vi "Fit Transform.vi"(7 "Type X":T1(ring), 8 "error in (no error)":errorcluster caption="entrée d'erreur (pas d'erreur)", 10 "X":string[][](array[string]), 11 "MissingIndicator.lvclass":refnum<class "MissingIndicator.lvclass">) -> (0 "error out":errorcluster caption="sortie d'erreur", 2 "Data":T2, 3 "MissingIndicator.lvclass":refnum<class "MissingIndicator.lvclass">)   [LabVIEW 2020, in "MissingIndicator.lvclass"]
doc: "Generate missing values indicator for X.\n\nReturns : \n\n- Xt : {ndarray or sparse matrix}, shape (n_samples, n_features) or (n_samples, n_features_with_missing)\nThe missing indicator for input data. The data type of Xt will be boolean."
uses:
  MissingIndicator.lvclass
  MissingIndicator.lvclass/MissingIndicator.ctl
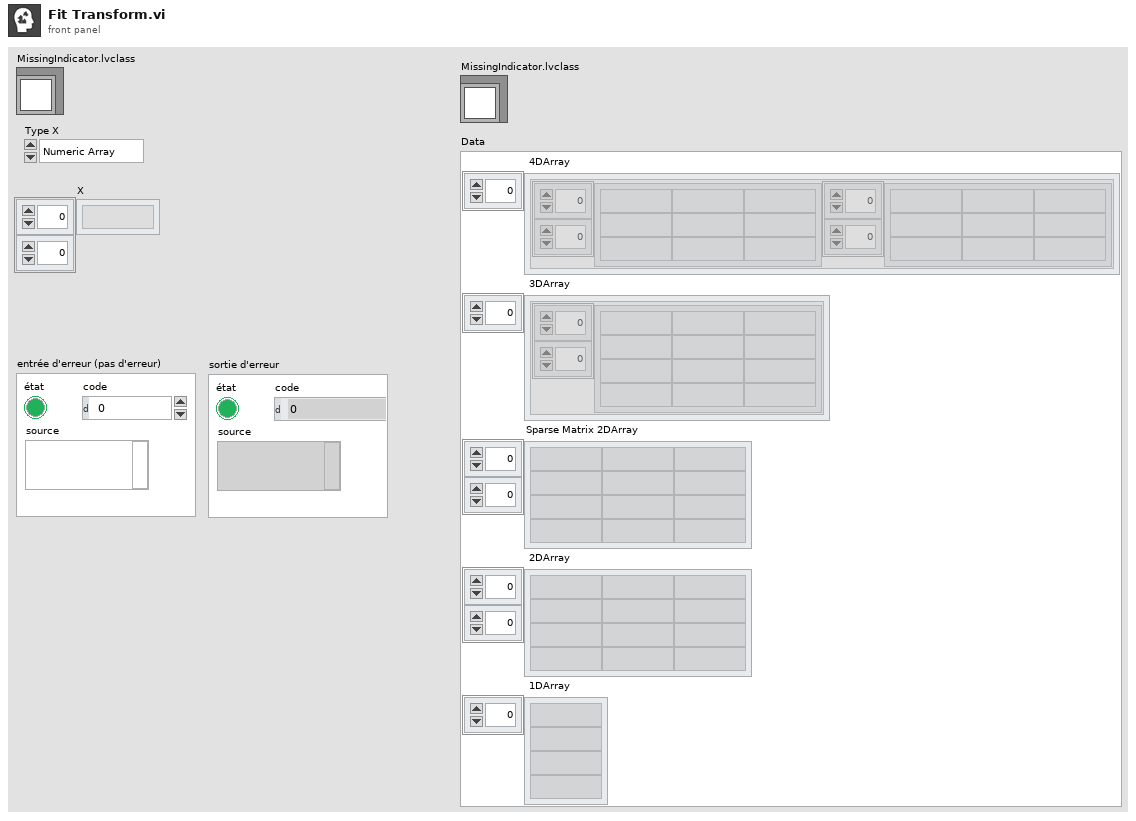
[diagram p1: front panel]
types:
  T1 = enum16{"Numeric Array", "String Array", "Sparse"}
  T2 = cluster{" 4DArray":cluster{"1":string[][], "2":string[][]}[], " 3DArray":cluster{"Tableau":string[][]}[], "Sparse Matrix 2DArray":string[][], " 2DArray":string[][], " 1DArray":string[]}
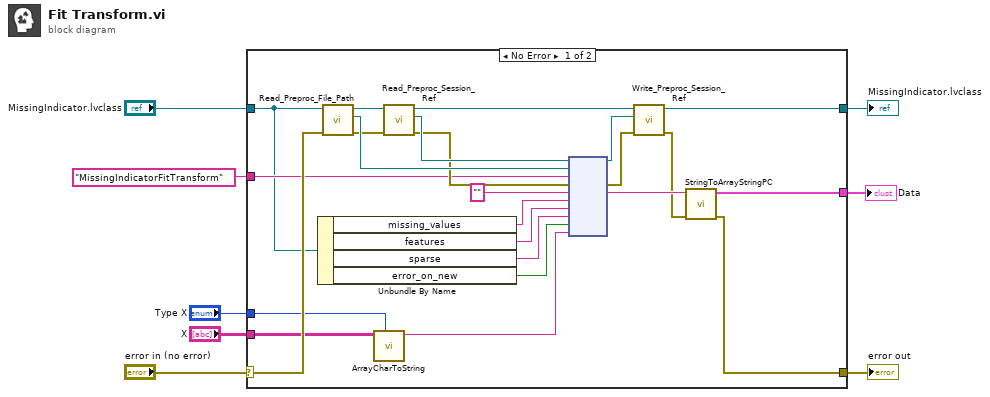
[diagram p0: block diagram]
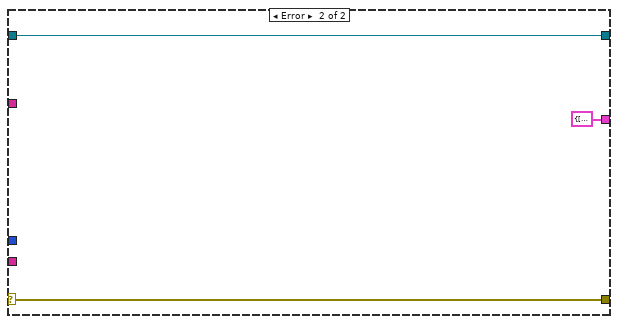
[diagram p2: hidden frame]
diagram:
  n1 = case shown="No Error" "error in (no error)" {
    selector: "error in (no error)" -> [w23 w35]
    tunnel: [w12 w35] -> w7
    tunnel: [w16 w34] -> w5
    tunnel: "MissingIndicator.lvclass" -> [w21 w34]
    tunnel: "MissingIndicatorFitTransform" ("Fonction") -> [w22 _]
    tunnel: [w14 T2 {" 4DArray"=[], " 3DArray"=[], "Sparse Matrix 2DArray"=[], " 2DArray"=[], " 1DArray"=[]} ("Data")] -> w2
    tunnel: "X" -> [w11 _]
    tunnel: "Type X" -> [w9 _]
    frame No Error {
      n2 = Unbundle By Name(w21) -> ("missing_values"=w20:string, "features"=w19:string, "sparse"=w18:string, "error_on_new"=w17:bool)
      n3 = call-dynamic "Read_Preproc_File_Path.vi"("error in (no error)"=w23, "Python in"=w21) -> ("error out"=w27:errorcluster, "File_Path"=w30:path, "Python out"=w32:refnum<class "MissingIndicator.lvclass">)  [unwired: 7 in]
      n4 = call "ArrayCharToString.vi"("Type"=w9, "TAB"=w11) -> ("Instruction"=w10:string)  [unwired: 9 in]
      n5 = call-dynamic "Read_Preproc_Session_Ref.vi"("error in (no error)"=w27, "Python in"=w32) -> ("error out"=w28:errorcluster, "Session_ref"=w29:refnum<k35>, "Python out"=w31:refnum<class "MissingIndicator.lvclass">)  [unwired: 7 in]
      n6 = node(w29, w30, w22, w28, "", w20, w19, w18, w17, w10) -> (w24:refnum<k35>, w26:errorcluster, w15:string)  [unwired: 5 in, 2 out]
      n7 = call-dynamic "Write_Preproc_Session_Ref.vi"("error in (no error)"=w26, "Session_ref"=w24, "Python in"=w31) -> ("error out"=w13:errorcluster, "Python out"=w16:refnum<class "MissingIndicator.lvclass">)  [unwired: 7 in]
      n8 = call "StringToArrayStringPC.vi"("sortie d'erreur"=w13, "Return value"=w15) -> ("sortie d'erreur"=w12:errorcluster, "Data"=w14:T2)  [unwired: 8 in]
    }
    frame Error {
    }
  }
  "error out" <- w7
  "MissingIndicator.lvclass" <- w5
  "Data" <- w2
